vi "Main Test.vi"(8 "error in (no error)":errorcluster, 10 "Generate Event?":bool) -> (0 "error out":errorcluster, 3 "Assert Message":string)   [LabVIEW 2017]
uses:
  Core/Assert API Components/Assert Event Actions.ctl
  Core/Assert API Components/Assert API Components.lvlib
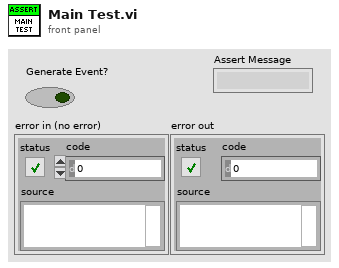
[diagram p1: front panel]
types:
  T1 = typedef "Assert API Components.lvlib/Assert Event Actions.ctl" = enum16{"Init", "Read", "Destroy"}
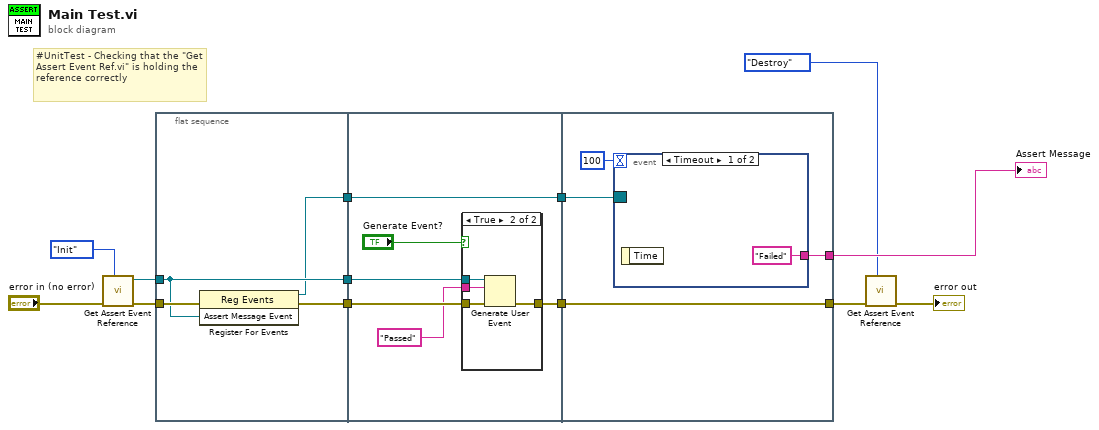
[diagram p0: block diagram]
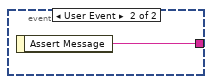
[diagram p3: hidden frame]
diagram:
  # "#UnitTest - Checking that the \"Get Assert Event Ref.vi\" is holding the reference correctly"
  n1 = call "Get Assert Event Reference.vi"("Action"=Assert_Event_Actions."Init", "error in (no error)"="error in (no error)") -> ("error out"=w10:errorcluster, "Assert Message Event"=w11:refnum<user-event>)  [unwired: 8 in]
  n2 = flat-sequence {
    tunnel: w11 -> [w15]
    tunnel: w10 -> [w17]
    tunnel: [w16] -> w9
    tunnel: [w15] -> w8
    tunnel: [w14] -> w6
    tunnel: w9 -> [w23]
    tunnel: w8 -> [w21]
    tunnel: [w22] -> w7
    tunnel: w6 -> [w19]
    tunnel: [w19] -> w5
    tunnel: [w32] -> w3
    tunnel: w7 -> [w32]
    tunnel: w5 -> [w30]
    tunnel: [w29] -> w4
    frame #0 {
      n3 = register-events(error in=w17, w15) -> (reference out=w14:refnum<event-registration>, error out=w16:errorcluster)  [unwired: 1 in]
    }
    frame #1 {
      n4 = case shown="True" "Generate Event?" {
        tunnel: w23 -> [w24 w28]
        tunnel: [w24 w27] -> w22
        tunnel: w21 -> [_ w26]
        tunnel: "Passed" ("event data") -> [_ w25]
        frame False {
        }
        frame True {
          n5 = Generate User Event(user event=w26, event data cluster=w25, error in=w28) -> (error out=w27:errorcluster)  [unwired: 1 in, 1 out]
        }
      }
    }
    frame #2 {
      n6 = event shown="[0] Timeout" {
        selector: w30 -> [_ _]
        dyn-events: _ -> [_ _]
        timeout: 100 -> [_ _]
        tunnel: ["Failed" ("Assert Message") w34] -> w29
        event Timeout {
          n7 = event-data() -> ()  [unwired: 1 in, 1 out]
        }
        event User Event {
          n8 = event-data() -> ("Assert Message"=w34:string)  [unwired: 1 in]
        }
      }
    }
  }
  n9 = call "Get Assert Event Reference.vi"("Action"=Assert_Event_Actions."Destroy", "error in (no error)"=w3) -> ("error out"=→"error out":errorcluster)  [unwired: 8 in, 1 out]
  "Assert Message" <- w4
